vi "Create.vi"(8 "error in (no error)":errorcluster, 10 "Source Code Poll":T1, 11 "Build Trigger":T2={"Day of Week"=enum."Everyday", "Hour"=1, "Enable?"=FALSE} {"Hour" min=0 max=23}) -> (0 "error out":errorcluster, 3 "Job Initialize out":refnum<class "Job Initialize.lvclass">)   [LabVIEW 2014, in "Job Initialize.lvclass"]
uses:
  Job Initialize.lvclass
  Controls/Cron String - STYP.ctl
  Controls/Source Code Control Selection - STYP.ctl
  Build Job/Build Job.lvclass/Build Job.ctl
  Job Initialize.lvclass/Job Initialize.ctl
  Build Job/Write Script Job Name.vi
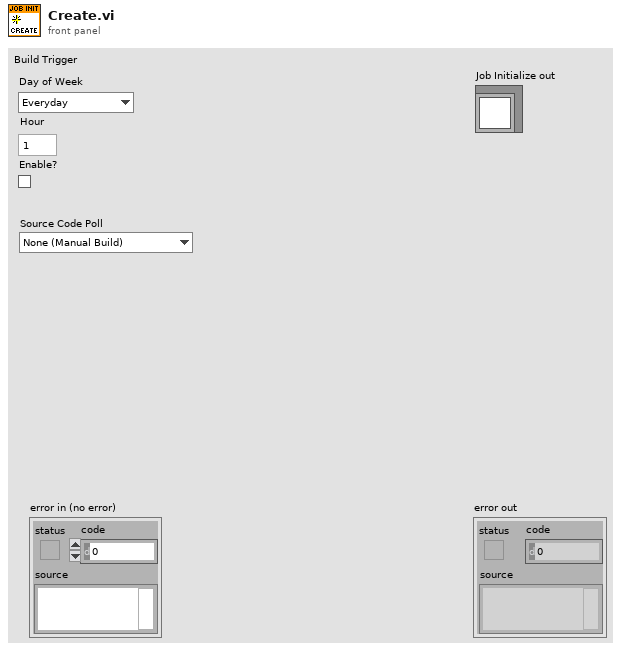
[diagram p1: front panel]
types:
  T1 = typedef "Source Code Control Selection - STYP.ctl" = enum16{"None (Manual Build)", "Every 15 Minutes", "Every 30 Minutes", "Every 45 Minutes", "Every Hour", "Every 2 Hours", "Everyday "}
  T2 = typedef "Cron String - STYP.ctl" = cluster{"Day of Week":enum16{"Everyday", "Sunday", "Monday", "Tuesday", "Wednesday", "Thursday", "Friday", "Saturday"}, "Hour":i32, "Enable?":bool}
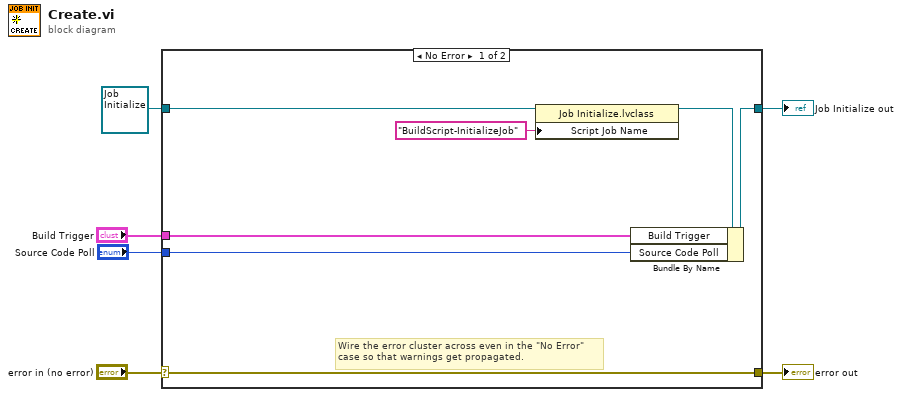
[diagram p0: block diagram]
diagram:
  n1 = case shown="No Error" "error in (no error)" {
    selector: "error in (no error)" -> [w13 w15]
    tunnel: [w13 w15] -> w5
    tunnel: [w10 w14] -> w3
    tunnel: refnum<class "Job Initialize.lvclass"> refnum ("Job Initialize in") -> [w12 w14]
    tunnel: "Build Trigger" -> [w9 _]
    tunnel: "Source Code Poll" -> [w7 _]
    frame No Error {
      # "Wire the error cluster across even in the \"No Error\"\ncase so that warnings get propagated."
      n2 = property class="Job Initialize.lvclass"(reference=w12, "Script Job Name"="BuildScript-InitializeJob") -> (reference out=w11:refnum<class "Job Initialize.lvclass">)  [unwired: 1 in, 1 out]
      n3 = Bundle By Name(cluster=w11, "Build Trigger"=w9, "Source Code Poll"=w7) -> (w10:refnum<class "Job Initialize.lvclass">)
    }
    frame Error {
    }
  }
  "error out" <- w5
  "Job Initialize out" <- w3
